vi "Do.vi"(8 "error in (no error)":errorcluster, 10 "Actor in":refnum<class "Actor.lvclass">, 11 "Lookup Value Msg":refnum<class "Lookup Value Msg.lvclass">) -> (0 "error out":errorcluster, 2 "Actor out":refnum<class "Actor.lvclass">)   [LabVIEW 2023, in "Nested.lvlib" / "Lookup Value Msg.lvclass"]
doc: "This VI delivers the message to the actor by calling the appropriate method(s) on the actor."
uses:
  Lookup Value Msg.lvclass
  <vilib>/ActorFramework/Actor/Actor.lvclass
  Lookup Value Msg.lvclass/Lookup Value Msg.ctl
  Nested/Nested.lvclass
  c:/dev/_r/4/eng/lv-core/lvpostprocessingd/lv_mc_x86_64/dist_i386/vi.lib/ActorFramework/Actor/Actor.lvclass
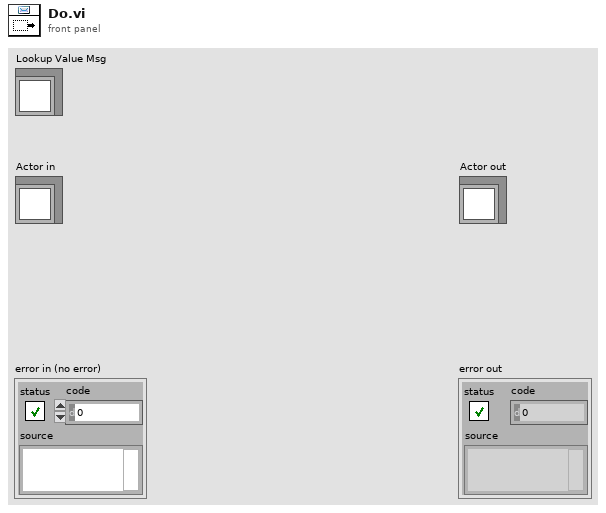
[diagram p1: front panel]
types:
  T1 = typedef "Nested.lvlib/Nested.lvclass/Named Value.ctl" = enum16{"e", "pi", "golden ratio"}
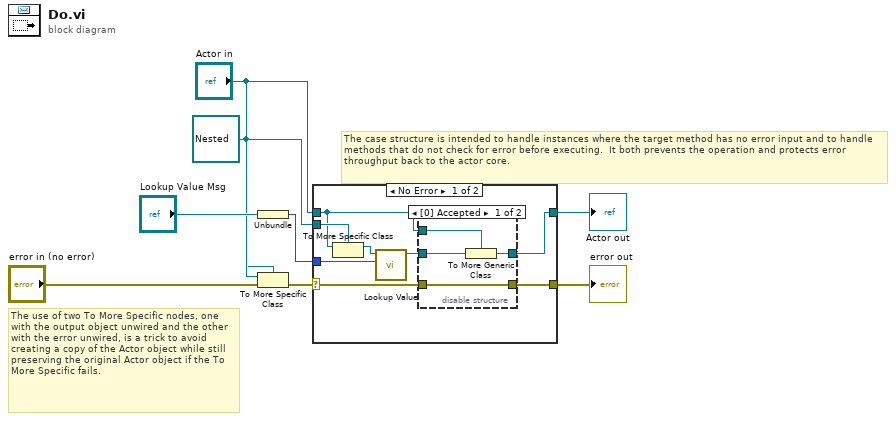
[diagram p0: block diagram]
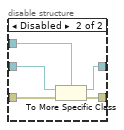
[diagram p2: hidden frame]
diagram:
  w2 = refnum<class "Nested.lvclass"> refnum ("Actor in")
  # "The use of two To More Specific nodes, one with the output object unwired and the other with the error unwired, is a trick to avoid creating a copy of the Actor object while still preserving the original Actor object if the To More Specific fails."
  # "The case structure is intended to handle instances where the target method has no error input and to handle methods that do not check for error before executing.  It both prevents the operation and protects error throughput back to the actor core."
  n1 = Unbundle("Lookup Value Msg") -> (w1:T1)
  n2 = To More Specific Class(target class=w2, reference="Actor in", error in="error in (no error)") -> (error out=w6:errorcluster)  [unwired: 1 out]
  n3 = case shown="No Error" w6 {
    selector: w6 -> [w16 w27]
    tunnel: [w13 w27] -> w5
    tunnel: [w12 w26] -> w4
    tunnel: "Actor in" -> [w10 w26]
    tunnel: w2 -> [w11 _]
    tunnel: w1 -> [w9 _]
    frame No Error {
      n4 = To More Specific Class(target class=w11, reference=w10) -> (specific class reference=w15:refnum<class "Nested.lvclass">)  [unwired: 1 in, 1 out]
      n5 = call "Lookup Value.vi"("named value"=w9, "Nested Actor in"=w15) -> ("Nested Actor out"=w14:refnum<class "Nested.lvclass">)  [unwired: 9 in]
      n6 = disable-structure shown="[0] Accepted" {
        disable-tunnel: [w19 w22] -> w12
        disable-tunnel: w14 -> [w18 w23]
        disable-tunnel: [w20 w24] -> w13
        disable-tunnel: w16 -> [w20 w25]
        disable-tunnel: w10 -> [w17 w21]
        frame Enabled {
          n7 = To More Generic Class(target class=w17, reference=w18) -> (generic class reference=w19:refnum<class "Actor.lvclass">)
        }
        frame Disabled {
          n8 = To More Specific Class(target class=w21, reference=w23, error in=w25) -> (specific class reference=w22:refnum<class "Actor.lvclass">, error out=w24:errorcluster)
        }
      }
    }
    frame Error {
      # "If type check fails, pass the original object out again."
    }
  }
  "error out" <- w5
  "Actor out" <- w4
